vi "Write Digital Output.vi"(8 "error in (no error)":errorcluster, 9 "State":bool, 10 "#Pin Digital Out":enum16{"DO-0", "DO-1", "DO-2", "DO-3"}(ring), 11 "VISA reference in":refnum<visa-resource-name>) -> (0 "error out":errorcluster, 2 "State dispare?":bool, 3 "VISA reference out":refnum<visa-resource-name>)   [LabVIEW 2020, in "Hardware DAQ.lvlib"]
uses:
  Hardware DAQ.lvlib
panel:
  out "resulting string":string
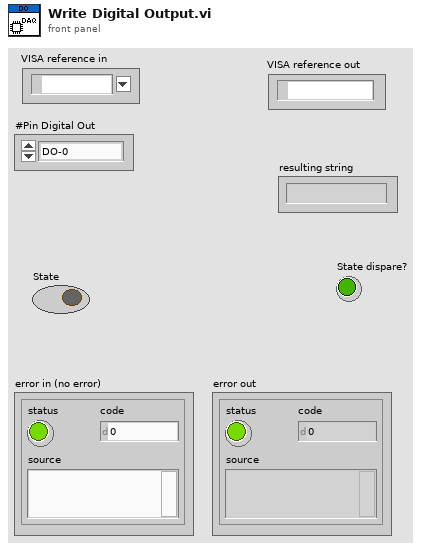
[diagram p1: front panel]
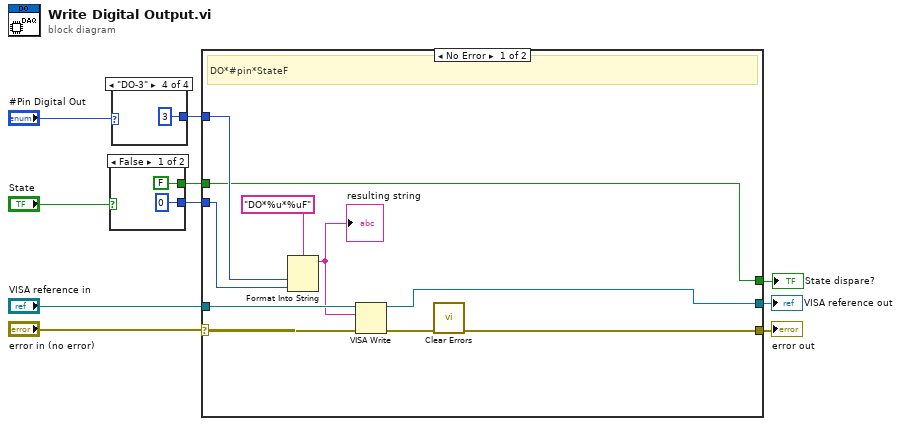
[diagram p0: block diagram]
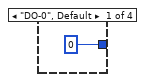
[diagram p2: hidden frame]
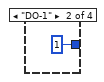
[diagram p3: hidden frame]
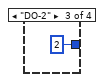
[diagram p4: hidden frame]
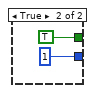
[diagram p5: hidden frame]
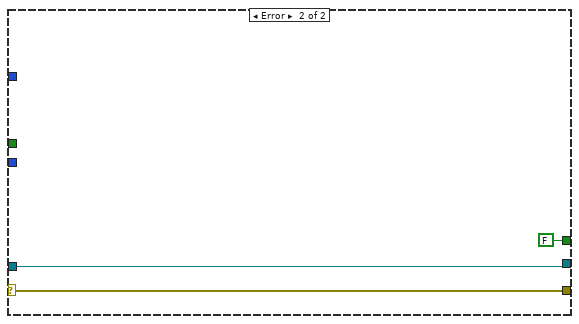
[diagram p6: hidden frame]
diagram:
  n1 = case shown="False" "State" {
    tunnel: [0 1] -> w5
    tunnel: [FALSE TRUE] -> w1
    frame False {
    }
    frame True {
    }
  }
  n2 = case shown="\"DO-3\"" "#Pin Digital Out" {
    tunnel: [0 1 2 3] -> w6
    frame "DO-0", Default {
    }
    frame "DO-1" {
    }
    frame "DO-2" {
    }
    frame "DO-3" {
    }
  }
  n3 = case shown="No Error" "error in (no error)" {
    selector: "error in (no error)" -> [w28 w31]
    tunnel: "VISA reference in" -> [w27 w30]
    tunnel: w6 -> [w26 _]
    tunnel: w5 -> [w25 _]
    tunnel: [w19 FALSE] -> w2
    tunnel: [w20 w31] -> w4
    tunnel: [w23 w30] -> w3
    tunnel: w1 -> [w19 _]
    frame No Error {
      # "DO*#pin*StateF"
      n4 = Format Into String(format string="DO*%u*%uF", w26, w25) -> (resulting string=w21:string)  [unwired: 2 in, 1 out]
      "resulting string" <- w21
      n5 = VISA Write(VISA resource name=w27, write buffer=w21, error in (no error)=w28) -> (VISA resource name out=w23:refnum<visa-resource-name>, error out=w24:errorcluster)  [unwired: 1 out]
      n6 = call <vilib>:"Clear Errors.vi"("error in (no error)"=w24) -> ("error out"=w20:errorcluster)  [unwired: 5 in, 1 out]
    }
    frame Error {
    }
  }
  "error out" <- w4
  "State dispare?" <- w2
  "VISA reference out" <- w3
